vi "Lake Shore 372 Configure Input and Acquire Reading.vi"() -> ()   [LabVIEW 2015]
doc: "This example shows how to configure an input's settings and resistance range and take a quadrature resistance reading. The Window input is used to set the percent full-scale of the reading limits. The user is also given the option of not configuring the input and taking a quadrature resistance reading only."
uses:
  <instrlib>/Lake Shore 372/Lake Shore 372.lvlib
panel:
  in  "Enable Channel (T: Enable)":bool=TRUE
  in  "Enable Filter (F: Off)":bool
  in  "Excitation  (T: On)":bool=TRUE
  in  "Autoscan (F: Off)":bool
  in  "Temperature Limit (0 Kelvin)":dbl min=0.0 max=1000.0 step=0.1
  in  "Preferred Units (2: Ohms)":u16(ring)=2 items=["Kelvin"=1, "Ohms"=2]
  in  "Resistance Range (17: 200 kOhm)":u16(ring)=17 items=["2.00 mOhm"=1, "6.32 mOhm"=2, "20.0 mOhm"=3, "63.2 mOhm"=4, "200 mOhm"=5, "632 mOhm"=6, "2.00 Ohm"=7, "6.32 Ohm"=8, "20.0 Ohm"=9, "63.2 Ohm"=10, "200 Ohm"=11, "632 Ohm"=12, "2.00 kOhm"=13, "6.32 kOhm"=14, "20.0 kOhm"=15, "63.2 kOhm"=16, "200 kOhm"=17, "632 kOhm"=18, "2.00 MOhm"=19, "6.32 MOhm"=20, "20.0 MOhm"=21, "63.2 MOhm"=22]
  in  "Autorange (0: OFF)":u16(ring) items=["Autorange off", "Autorange Current", "ROX 102B Autorange"]
  in  "Excitation Range (5: 200 uV / 100 pA)":u16(ring)=5 items=["2.00 uV / 1.00 pA"=1, "6.32 uV / 3.16 pA"=2, "20.0 uV / 10.0 pA"=3, "63.2 uV / 31.6 pA"=4, "200 uV / 100 pA"=5, "632 uV / 316 pA"=6, "2.00 mV / 1.00 nA"=7, "6.32 mV / 3.16 nA"=8, "20.0 mV / 10.0 nA"=9, "63.2 mV / 31.6 nA"=10, "200 mV / 100 nA"=11, "632 mV / 316 nA"=12, "1.00 uA"=13, "3.16 uA"=14, "10.0 uA"=15, "31.6 uA"=16, "100 uA"=17, "316 uA"=18, "1.00 mA"=19, "3.16 mA"=20, "10.0 mA"=21, "31.6 mA"=22]
  in  "Excitation Mode (0: Voltage)":u16(ring) items=["Voltage", "Current"]
  in  "Window (40% FS)":i32=40 min=1 max=80 step=1
  in  "Settle Time (10 sec)":i32=10 min=1 max=200 step=1
  in  "Curve Number (0)":i32 min=0 max=59 step=1
  in  "Change Pause Time (3)":dbl=3.0 min=3.0 max=200.0 step=1.0
  in  "Input Name":string
  in  "Temperature Coefficient (1: Negative)":u16(ring)=1 items=["Negative"=1, "Positive"=2]
  in  "Scan Dwell Time (10)":dbl=10.0 min=1.0 max=200.0 step=1.0
  in  "Channel (1)":u16(ring)=1 items=["All Channels (0)", "1", "2", "3", "4", "5", "6", "7", "8", "9", "10", "11", "12", "13", "14", "15", "16", "A (Control Input)"]
  out "Resistance Reading":dbl min=0.0 max=63200000.0 step=1e-05 format="%^.5e"
  out "Quadrature Reading":dbl min=0.0 max=0.01 step=1e-05 format="%^.5e"
  out "Power Reading (W)":dbl min=0.0 max=0.01 step=1e-05 format="%^.5e"
  out "Kelvin Reading":dbl min=0.0 max=1000.0 step=1e-05 format="%^.5e"
  in  "Baud Rate (3: 57600)":i32(ring)=3 items=["300", "1200", "9600", "57600 (USB Only)"]
  in  "VISA resource name":refnum<visa-resource-name>
  in  "Configure (False)":bool
  # "(c) 2015 Advint LLC. ALL RIGHTS RESERVED."
  # "Input Channel Parameters"
  # "Channel Filter Parameters"
  # "Input Type Parameters"
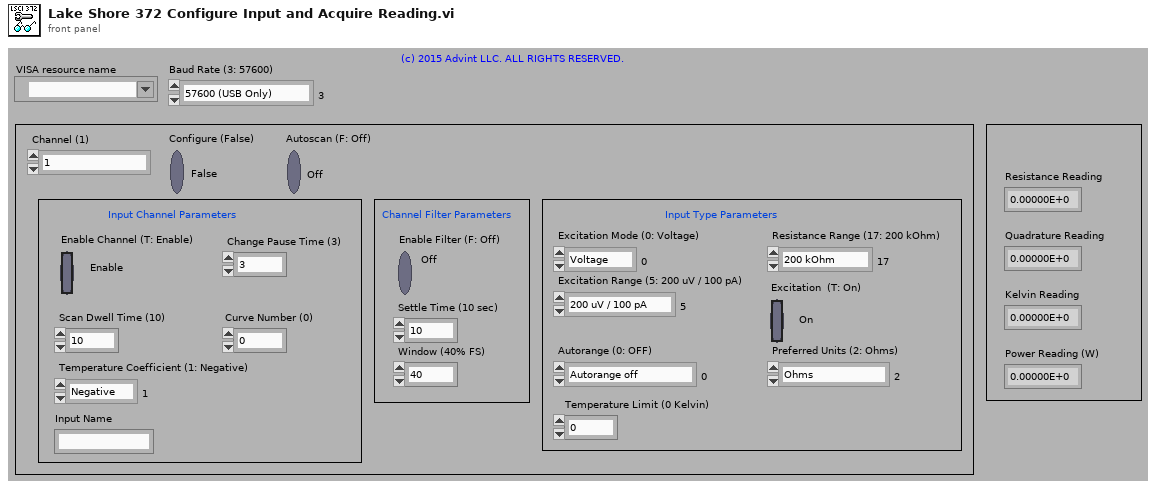
[diagram p1: front panel]
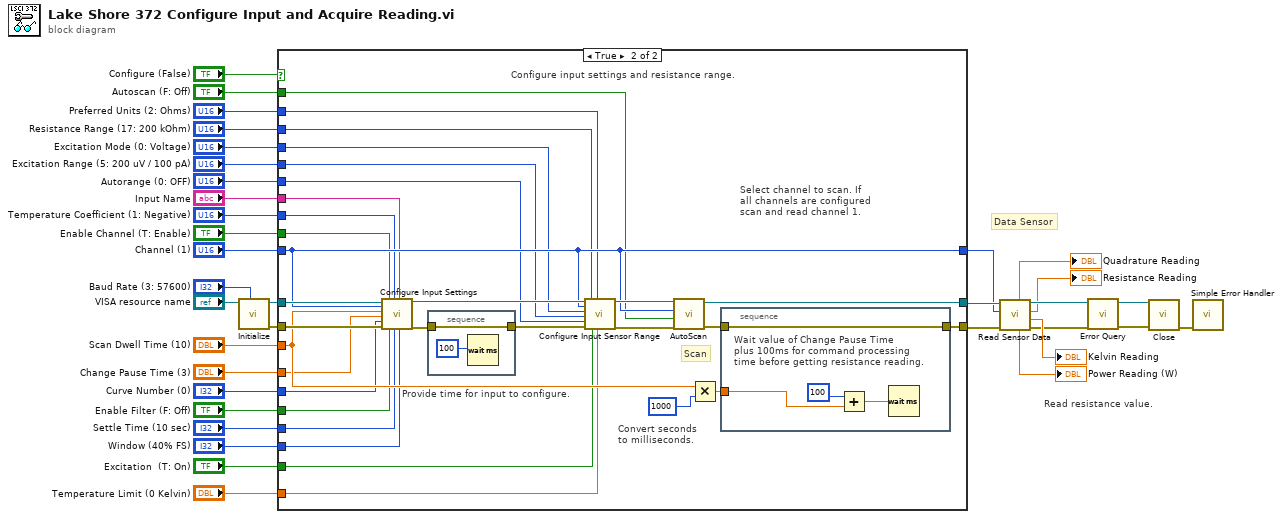
[diagram p0: block diagram]
diagram:
  # "Data Sensor"
  # "Read resistance value."
  n1 = call <instrlib>:"Initialize.vi"("Baud Rate (3: 57600)"="Baud Rate (3: 57600)", "VISA resource name"="VISA resource name") -> ("error out"=w34:errorcluster, "VISA resource name out"=w35:refnum<visa-resource-name>)  [unwired: 8 in]
  n2 = case shown="True" "Configure (False)" {
    tunnel: w34 -> [w37 w68]
    tunnel: w35 -> [w38 w67]
    tunnel: [w37 w66] -> w32
    tunnel: [w38 w62] -> w31
    tunnel: [w36 w56] -> w18
    tunnel: "Channel (1)" -> [w36 w56]
    tunnel: "Autoscan (F: Off)" -> [_ w48]
    tunnel: "Scan Dwell Time (10)" -> [_ w55]
    tunnel: "Change Pause Time (3)" -> [_ w54]
    tunnel: "Curve Number (0)" -> [_ w53]
    tunnel: "Window (40% FS)" -> [_ w52]
    tunnel: "Settle Time (10 sec)" -> [_ w51]
    tunnel: "Enable Filter (F: Off)" -> [_ w47]
    tunnel: "Enable Channel (T: Enable)" -> [_ w46]
    tunnel: "Temperature Coefficient (1: Negative)" -> [_ w50]
    tunnel: "Input Name" -> [_ w49]
    tunnel: "Autorange (0: OFF)" -> [_ w42]
    tunnel: "Excitation Range (5: 200 uV / 100 pA)" -> [_ w41]
    tunnel: "Excitation Mode (0: Voltage)" -> [_ w40]
    tunnel: "Resistance Range (17: 200 kOhm)" -> [_ w39]
    tunnel: "Preferred Units (2: Ohms)" -> [_ w43]
    tunnel: "Temperature Limit (0 Kelvin)" -> [_ w44]
    tunnel: "Excitation  (T: On)" -> [_ w45]
    frame False {
      # "Do not configure input settings and resistance range."
      # "Select channel to scan. If\nall channels are selected\nscan and read channel 1."
    }
    frame True {
      # "Scan"
      # "Provide time for input to configure."
      # "Select channel to scan. If\nall channels are configured\nscan and read channel 1."
      # "Configure input settings and resistance range."
      # "Convert seconds to milliseconds."
      n3 = call <instrlib>:"Configure Input Settings.vi"("VISA resource name"=w67, "Channel (1)"=w56, "Scan Dwell Time (10)"=w55, "Change Pause Time (3)"=w54, "Curve Number (0)"=w53, "error in (no error)"=w68, "Enable Channel (T: Enable)"=w46, "Enable Filter (F: Off)"=w47, "Temperature Coefficient (1: Negative)"=w50, "Settle Time (10 sec)"=w51, "Input Name"=w49, "Window (40% FS)"=w52) -> ("VISA resource name out"=w58:refnum<visa-resource-name>, "error out"=w63:errorcluster)  [unwired: 6 in]
      n4 = stacked-sequence {
        tunnel: w63 -> [w69]
        tunnel: [w69] -> w60
        frame #0 {
          n5 = Wait (ms)(milliseconds to wait=100) -> ()  [unwired: 1 out]
        }
      }
      n6 = call <instrlib>:"Configure Input Sensor Range.vi"("VISA resource name"=w58, "Channel (1)"=w56, "Excitation Mode (0: Voltage)"=w40, "Excitation Range (5: 200 uV / 100 pA)"=w41, "Autorange (0: Autorange off)"=w42, "error in (no error)"=w60, "Resistance Range (17: 200 kOhm)"=w39, "Excitation  (T: On)"=w45, "Preferred Units (2: Ohms)"=w43, "Temperature Limit (0 Kelvin)"=w44) -> ("VISA resource name out"=w57:refnum<visa-resource-name>, "error out"=w59:errorcluster)  [unwired: 8 in]
      n7 = call <instrlib>:"AutoScan.vi"("error in (no error)"=w59, "Autoscan (F: Off)"=w48, "Channel (1:1)"=w56, "VISA resource name"=w57) -> ("error out"=w61:errorcluster, "VISA resource name out"=w62:refnum<visa-resource-name>)  [unwired: 6 in]
      n8 = Multiply(x=w55, y=1000) -> (x*y=w64:dbl)
      n9 = stacked-sequence {
        tunnel: w61 -> [w74]
        tunnel: [w74] -> w66
        tunnel: w64 -> [w72]
        frame #0 {
          # "Wait value of Change Pause Time  \nplus 100ms for command processing \ntime before getting resistance reading."
          n10 = Add(x=100, y=w72) -> (x+y=w71:dbl)
          n11 = Wait (ms)(milliseconds to wait=w71) -> ()  [unwired: 1 out]
        }
      }
    }
  }
  n12 = call <instrlib>:"Read Sensor Data.vi"("error in (no error)"=w32, "Channel (1:1)"=w18, "VISA resource name"=w31) -> ("error out"=w25:errorcluster, "Kelvin Reading"=→"Kelvin Reading":dbl, "Resistance Reading"=→"Resistance Reading":dbl, "VISA resource name out"=w24:refnum<visa-resource-name>, "Power Reading"=→"Power Reading (W)":dbl, "Quadrature Reading"=→"Quadrature Reading":dbl)  [unwired: 3 in]
  n13 = call <instrlib>:"Error Query.vi"("error in (no error)"=w25, "VISA resource name"=w24) -> ("error out"=w22:errorcluster, "VISA resource name out"=w23:refnum<visa-resource-name>)  [unwired: 7 in, 1 out]
  n14 = call <instrlib>:"Close.vi"("error in (no error)"=w22, "VISA resource name"=w23) -> ("error out"=w29:errorcluster)  [unwired: 9 in]
  n15 = call <vilib>:"Simple Error Handler.vi"("error in (no error)"=w29) -> ()  [unwired: 4 in, 5 out]
